vi "Oblicznie_wektora_przestrzennego.vi"(9 "I_C":dbl[](array[numeric]), 10 "I_B":dbl[](array[numeric]), 11 "I_A":dbl[](array[numeric])) -> (0 "i_p":dbl[](array[numeric]), 3 "i_alfa, i_beta":cluster{dbl[], dbl[]})   [LabVIEW 2018]
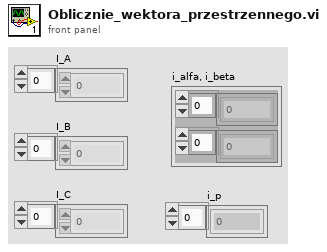
[diagram p1: front panel]
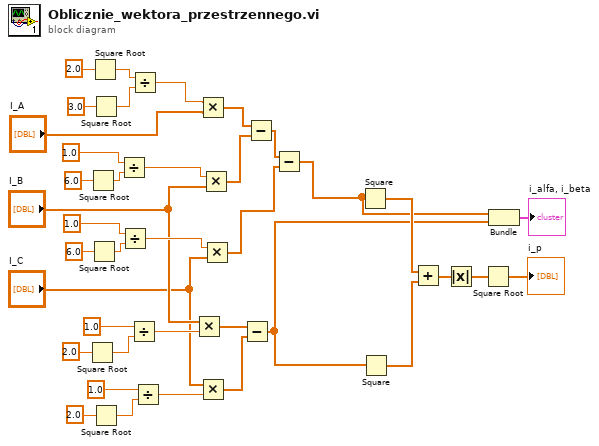
[diagram p0: block diagram]
diagram:
  n1 = Square Root(x=2.0) -> (sqrt(x)=w19:dbl)
  n2 = Square Root(x=6.0) -> (sqrt(x)=w26:dbl)
  n3 = Square Root(x=6.0) -> (sqrt(x)=w35:dbl)
  n4 = Square Root(x=2.0) -> (sqrt(x)=w23:dbl)
  n5 = Square Root(x=3.0) -> (sqrt(x)=w24:dbl)
  n6 = Square Root(x=2.0) -> (sqrt(x)=w13:dbl)
  n7 = Divide(x=1.0, y=w26) -> (x/y=w32:dbl)
  n8 = Divide(x=1.0, y=w35) -> (x/y=w37:dbl)
  n9 = Divide(x=1.0, y=w19) -> (x/y=w17:dbl)
  n10 = Divide(x=w23, y=w24) -> (x/y=w29:dbl)
  n11 = Divide(x=1.0, y=w13) -> (x/y=w11:dbl)
  n12 = Multiply(x="I_B", y=w17) -> (x*y=w15:dbl[])
  n13 = Multiply(x=w29, y="I_A") -> (x*y=w31:dbl[])
  n14 = Multiply(x="I_C", y=w11) -> (x*y=w9:dbl[])
  n15 = Multiply(x=w32, y="I_B") -> (x*y=w33:dbl[])
  n16 = Multiply(x=w37, y="I_C") -> (x*y=w38:dbl[])
  n17 = Subtract(x=w15, y=w9) -> (x-y=w2:dbl[])
  n18 = Subtract(x=w31, y=w33) -> (x-y=w28:dbl[])
  n19 = Subtract(x=w28, y=w38) -> (x-y=w3:dbl[])
  n20 = Square(x=w3) -> (x^2=w8:dbl[])
  n21 = Square(x=w2) -> (x^2=w7:dbl[])
  n22 = Add(x=w8, y=w7) -> (x+y=w6:dbl[])
  n23 = Absolute Value(x=w6) -> (abs(x)=w5:dbl[])
  n24 = Square Root(x=w5) -> (sqrt(x)=→"i_p":dbl[])
  n25 = Bundle(w3, w2) -> (→"i_alfa, i_beta":cluster{dbl[], dbl[]})  [unwired: 1 in]
